vi "Saver.vi"(8 "error in":errorcluster, 11 "TEXT":string) -> (0 "error out":errorcluster)   [LabVIEW 2023]
doc: "Dieses VI loggt den Status des Programmes mit.\nErstellt: Batarilo Marino \n01.10.2025"
panel:
  out "time string":string
  out "date string":string
  out "Application Directory":path
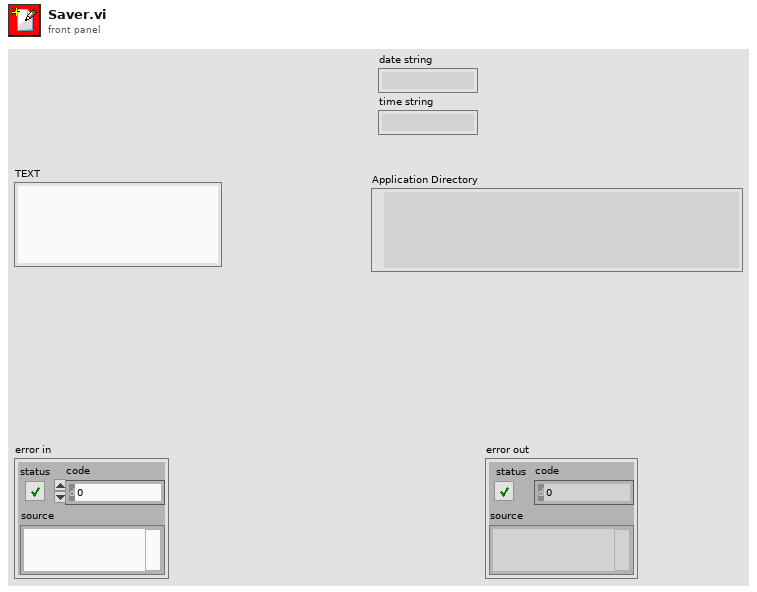
[diagram p1: front panel]
types:
  T1 = enum16{"open", "replace", "create", "open or create", "replace or create", "replace or create with confirmation"}
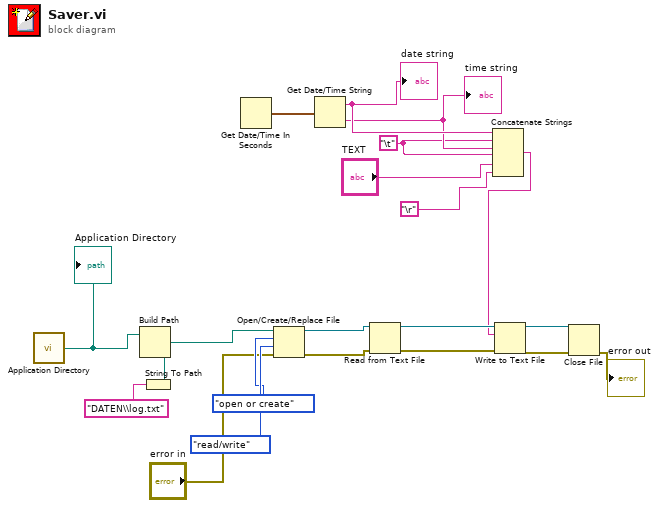
[diagram p0: block diagram]
diagram:
  w5 = "\t"
  n1 = call <vilib>:"Application Directory.vi"() -> ("Application Directory"=w21:path)
  "Application Directory" <- w21
  n2 = String To Path(string="DATEN\\log.txt") -> (path=w16:path)
  n3 = Build Path(base path=w21, name or relative path=w16) -> (appended path=w20:path)
  n4 = Get Date/Time In Seconds() -> (seconds since 1Jan1904=w8:timestamp)
  n5 = Open/Create/Replace File(file path (use dialog)=w20, error in="error in", operation (0:open)=T1."open or create", access (0:read/write)=enum16{"read/write", "read-only", "write-only"}."read/write") -> (refnum out=w15:refnum<file>, error out=w10:errorcluster)  [unwired: 2 in, 1 out]
  n6 = Get Date/Time String(seconds (now)=w8) -> (date string=w7:string, time string=w6:string)  [unwired: 2 in]
  "date string" <- w7
  "time string" <- w6
  n7 = Read from Text File(file (use dialog)=w15, error in=w10) -> (refnum out=w14:refnum<file>, error out=w11:errorcluster)  [unwired: 2 in, 2 out]
  n8 = Concatenate Strings(w7, w5, w6, w5, "TEXT", "\r") -> (w9:string)
  n9 = Write to Text File(file (use dialog)=w14, text=w9, error in=w11) -> (refnum out=w13:refnum<file>, error out=w12:errorcluster)  [unwired: 1 in, 1 out]
  n10 = Close File(refnum=w13, error in=w12) -> (error out=→"error out":errorcluster)  [unwired: 1 out]
